vi "Global.vi"() -> ()   [LabVIEW 2020, in "Ballard 1553 Shared.lvlib"]
uses:
  Ballard 1553 Shared.lvlib
panel:
  in  "Tab Control":T1(tab)
  in  "Mode Code Section GUID":string="25e74143-3f22-4765-951b-e0255ac02f03"
  in  "Command Channels Section GUID":string="262c77c2-cd1e-4f56-ad53-4530960403b6"
  in  "BC Acyclic Frame Trigger Channel GUID":string="c5d03647-e2a2-4aa7-8b94-b69019d44c40"
  in  "Remote Terminal Status Word":string="1f61d0e0-e62d-4b27-95bd-3fdf789bbd0f"
  in  "Remote Terminal subAddress GUID":string="d1c4e349-acfd-4088-bf4d-ea1112e00b30"
  in  "Remote Terminal GUID":string="8b675cd2-9797-4263-b482-91598d9c6e7a"
  in  "Command Channel GUID":string="42c75256-e247-4fc5-9ed9-70c38e6c1705"
  in  "Status Channel GUID":string="51bb2b0d-84b0-4f68-8c96-70c74a1d4fc0"
  in  "Data Word Channel GUID":string="26cd04cf-934e-4ac4-8a82-5f7f40e7f840"
  in  "Data Words Section GUID":string="ea34343c-a380-4f25-833d-9a3726be6ed2"
  in  "Message Section GUID":string="d8b532bb-7481-48a0-bd8b-cd4e7607613f"
  in  "Timestamp GUID":string="93a38d79-2c39-4060-8504-93f4bbab327b"
  in  "Bus Controller Page GUID":string="11c6c936-cda4-4307-8188-503fb6a96b76"
  in  "Channel Page GUID":string="ea467fec-7216-4c5b-a739-9b555c5a9c2a"
  in  "Status Section GUID":string="d7eafe26-ed14-47ff-9bb7-6b94adfafad3"
  in  "Static Chan GUID":string="0647d62a-fc3c-4842-83dd-8dc02dd29b16"
  in  "MainDisabled":string="2f907296-a531-4167-811c-f760cafa0ba4"
  in  "MainEnabled":string="9d335017-4496-4762-9bed-0bac8b9be886"
  in  "BC.Command Channel.Acyclic Frame.Name":string="BC.Command Channel.Acyclic Frame.Name"
  in  "Remote Terminal.modeCode.ID":string="Remote Terminal.modeCode.ID"
  in  "RT.modeCode Section":string="Mode Codes"
  in  "Remote Terminal.SA.ID":string="Remote Terminal.SA.ID"
  in  "RT.SA.Name Direction Postfix String Tx":string="(Tx)"
  in  "RT.SA.Name Direction Postfix String Rx":string="(Rx)"
  in  "BC.Command Channel.Acyclic Frame Prefix":string="Trigger"
  in  "Word Error":string="Word Error Counter"
  in  "Parity Error":string="Parity Error Counter"
  in  "Manchester Error":string="Manchester Error Counter"
  in  "Improper Number of Data Words Error":string="Improper Number of Data Words Error Counter"
  in  "Wrong Sync Error":string="Wrong Sync Error Counter"
  in  "General Protocol Error":string="General Protocol Error Counter"
  in  "Monitor - Error Counter":string="Monitor - Error Counter"
  in  "Bus Controller.Message.Status Word Receive RT":string="Status Word (Rx)"
  in  "Bus Controller.Message.Status Word Transmit RT":string="Status Word (Tx)"
  in  "Remote Terminal.Raw Data Words Section":string="Data Words"
  in  "RT.Status Channel":string="Status Channel"
  in  "RT.Command Channel.Stop RT":string="Stop RT"
  in  "RT.Command Channel.Start RT":string="Start RT"
  in  "RT.Command Channels Section":string="Command Channels"
  in  "Remote Terminal":string="Remote Terminal"
  in  "BC.Command Channel.Stop BC":string="Stop BC"
  in  "BC.Command Channel.Start BC":string="Start BC"
  in  "BC.Command Channels Section":string="Command Channels"
  in  "Timestamp Channels":string="Timestamp"
  in  "Bus Controller.Message.Status Word":string="Status Word"
  in  "Data Words Section":string="Data Words"
  in  "Bus Controller.ID":string="Bus Controller.ID"
  in  "Bus Controller.name":string="Bus Controller.name"
  in  "Bus Controller":string="Bus Controller"
  in  "Message.ParamID":string="Message.ParamID"
  in  "Remote Terminal.modeCode.Direction":string="Remote Terminal.modeCore Remote Terminal.modeCode.Direction"
  in  "Remote Terminal.modeCode.Number":string="Remote Terminal.modeCode.NumbeRemote Terminal.modeCode.Number"
  in  "Message.ID":string="Message.ID"
  in  "Unconfigured Frames Counter":string="Unconfigured Frames Counter"
  in  "Remote Terminal.Raw Data Word":string="Word"
  in  "Remote Terminal.Terminal direction":string="Remote Terminal.Terminal direction"
  in  "Remote Terminal.Terminal Sub-Address":string="Remote Terminal.Terminal SubAddress"
  in  "Remote Terminal.rtMode":string="Remote Terminal.rtMode"
  in  "Remote Terminal.Terminal Address":string="Remote Terminal.Terminal Address"
  in  "Frames Timestamp Channels":string="Frames Timestamp Channels"
  in  "Message.CWD2":string="Message.CWD2"
  in  "Message.CWD1":string="Message.CWD1"
  in  "Message.messageType":string="Message.messageType"
  in  "Channel #":string="Channel #"
  in  "ParametersFileHash":string="ParametersFileHash"
  in  "Win Parameters File Path":string="Win Parameters File Path"
  in  "DBHash":string="DBHash"
  in  "Win File Path":string="Win File Path"
  in  "Inline Read Time":string="Inline Read Time"
  in  "Asynchronous LoopTime":string="Asynchronous Loop Time"
  in  "Inline Write Time":string="Inline Write Time"
  in  "Inline Error Code":string="Inline Error Code"
  in  "Status Section":string="Status"
  in  "PXI Slot Number":string="PXI Slot Number"
  in  "Initialization Method":string="Initialization Method"
  in  "core number":string="core number"
  in  "card number":string="card number"
  in  "Load Parameters File Action VI - Message1":string="There is no Hardware Configuration loaded. You cannot load a Parameters File."
  in  "Load Parameters File Action VI - Message2":string="There is already a Parameters File loaded. Click OK to continue and all existing System Mappings (connecting Parameters Channels) will be lost. Click Cancel to stop load operation."
  in  "Status Channels Section Description":string="This Section lists MIL-1553 Custom Device Status Channels."
  in  "Custom Device Main Page Description.":string="This Custom Device supports MIL-1553 boards from Ballard.\n\nIt's important to note:\n- Only supported hardware are the \"NI-Keyed boards only\", product Part Number should have the form: “LV-###-###-###.”\n- Supported hardware must be Multi-Function model (Single-Function model NOT supported)."
  in  "Unconfigured Frame Channel Counter Status Channel Description":string="This Channel is incremented as soon as a frame is received but it's not listed in the XML Configuration.\n\nIt's a U32 (Unsigned 32 Bits) counter shared between all Channels from Core configured. If Terminal Count (TC) is reached (0xFFFFFFFF), then value rolls off to 0."
  in  "Inline Write Time Status Channel Description":string="This Channel gives the Execution Time Duration (in us) for the Inline Write Case part of the MIL-1553 Custom Device for Ballard boards."
  in  "Inline Read Time Status Channel Description":string="This Channel gives the Execution Time Duration (in us) for the Inline Read Case part of the MIL-1553 Custom Device for Ballard boards."
  in  "Inline Error Code Status Channel Description":string="This Channel gives the last Error Code for Inline part of the MIL-1553 Custom Device for Ballard boards. 0 means no error."
  in  "Asynchronous Loop Time Status Channel Description":string="This Channel gives the Execution Time Duration (in us) for the Asynchronous Loop part of the MIL-1553 Custom Device for Ballard boards."
  in  "On Save Action VI - Message1":string="Error. Several Arinc-429 Ballard Custom Device instances have same combination of Initialization Method: PXI Slot Number or Card Number and Core Number. Deployment won't complete successfully."
  in  "Load Database - Message1":string="Warning. At least another Custom Device instance is configured with same Hardware Configuration File. It is a supported use-case and more for user's attention."
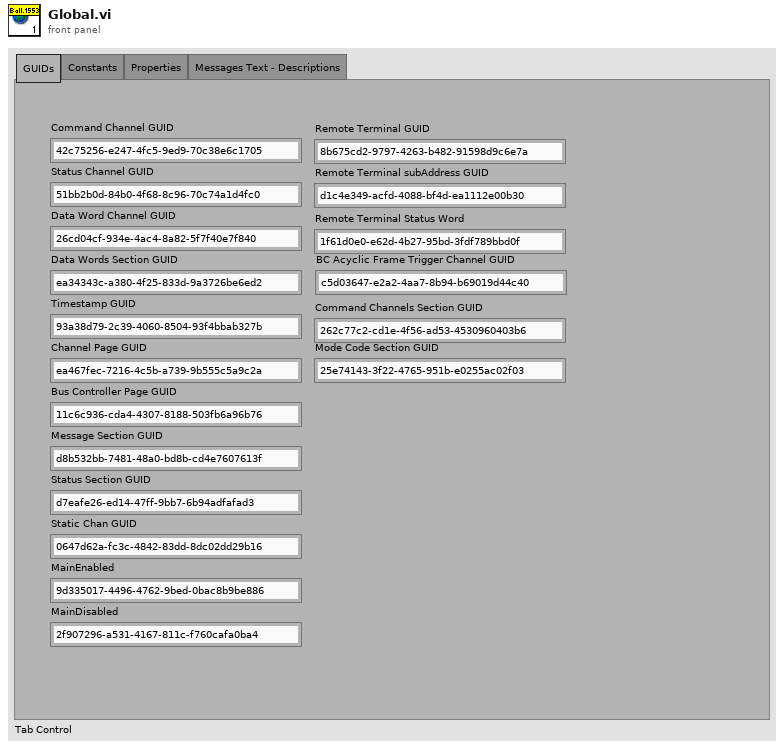
[diagram p1: front panel]
types:
  T1 = enum32{"GUIDs", "Constants", "Properties", "Messages Text - Descriptions"}
diagram:
